vi "FTW-TestExecutive-Core_OnStepChange.vi"(0 "FTW-TestExecutive-Core In":refnum<class "FTW-TestExecutive-Core.lvclass">, 11 "error in":errorcluster) -> (4 "FTW-TestExecutive-Core Out":refnum<class "FTW-TestExecutive-Core.lvclass">, 15 "error out":errorcluster)   [LabVIEW 2018, in "FTW-TestExecutive-Core.lvclass"]
uses:
  FTW-TestExecutive-Core.lvclass
  C:/Jobs/Featherweight/featherweight-2018/source/actor/Instance/FTW-ActorInstance.lvclass
  JSON/FTW-JSON-JoinMode.ctl
  FTW-TestExecutive-Core.lvclass/FTW-TestExecutive-Core.ctl
  3b20a742-de1c-4da6-9b17-d9e03c781a80.vi
  3b20a742-de1c-4da6-9b17-d9e03c781a80.vi/3871bf52-889f-4dbc-808d-62ab8c5fbf90.vi
  container/FTW-Container-FromVariant.vi
  container/FTW-Container-New-FromContainer.vi
  JSON/FTW-JSON-SerializeAndDestroy.vi
  Instance/FTW-ActorInstance.lvclass
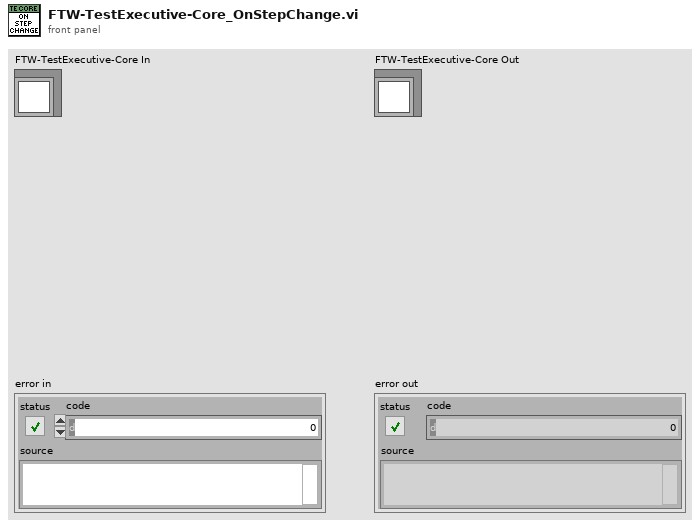
[diagram p1: front panel]
types:
  T1 = typedef "FTW-JSON-JoinMode.ctl" = enum32{"Upsert", "Update Only", "Insert Only"}
  T2 = typedef "FTW-TestExecutive-Step.ctl" = cluster{"Name":string, "Type":string, "Config":string, "Elapsed Time":dbl, "Passed":bool, "State":T3, "Results":T4}
  T3 = typedef "FTW-TestExecutive-Step-State.ctl" = enum8{"None", "Failed", "Passed", "Timed out", "Aborted"}
  T4 = typedef "FTW-TestExecutive-Results.ctl" = cluster{"Start Time":timestamp, "Elapsed Time":dbl, "Passed":bool, "Additional Results":string}
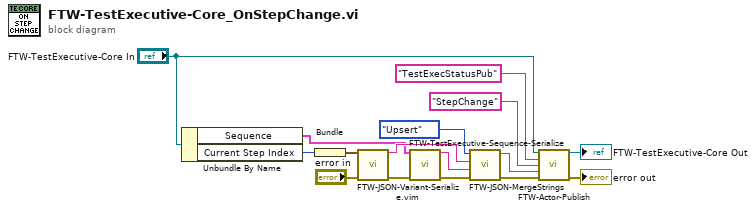
[diagram p0: block diagram]
diagram:
  n1 = Unbundle By Name("FTW-TestExecutive-Core In") -> ("Sequence"=w3:T2[], "Current Step Index"=w4:i32)
  n2 = Bundle("Current Step Index"=w4) -> (w6:cluster{"Current Step Index":i32})  [unwired: 1 in]
  n3 = call "FTW-JSON-Variant-Serialize.vim"("Variant"=w6, "error in"="error in") -> ("JSON String"=w7:string, "error out"=w10:errorcluster)  [unwired: 12 in]
  n4 = call "FTW-TestExecutive-Sequence-Serialize.vi"("Sequence"=w3, "error in"=w10) -> ("JSON"=w8:string, "error out"=w11:errorcluster)  [unwired: 12 in]
  n5 = call "FTW-JSON-MergeStrings.vi"("error in (no error)"=w11, "Initial JSON String (\"\")"=w8, "JSON string to merge (\"\")"=w7, "Update Mode (0: Upsert)"=FTW-JSON-JoinMode."Upsert") -> ("error out"=w2:errorcluster, "Merged JSON String (UTF-8)"=w1:string)  [unwired: 6 in]
  n6 = call "FTW-Actor-Publish.vi"("FTW-ActorExtended In"="FTW-TestExecutive-Core In", "Publisher Name"="TestExecStatusPub", "Message Header"="StepChange", "Message Body"=w1, "error in"=w2) -> ("FTW-ActorExtended Out"=→"FTW-TestExecutive-Core Out":refnum<class "FTW-TestExecutive-Core.lvclass">, "error out"=→"error out":errorcluster)  [unwired: 9 in]
